vi "HFRR ADV v031 new software.vi"() -> ()   [LabVIEW 2025] (continued)
                    tunnel: w3949 -> [w3955 w3956 _ _ w3957 w3958 w3959 w3961 w3963 w3965 w3967 w3969 w3971 w3973 _]
                    tunnel: w3948 -> [_ _ _ _ _ _ _ _ _ _ _ _ _ _ _]
                    frame 0 {
                      "TITTLE" <- w3955
                    }
                    frame 1 {
                      "Sample ID" <- w3956
                    }
                    frame 2 {
                    }
                    frame 3 {
                    }
                    frame 4 {
                      "Test Date" <- w3957
                    }
                    frame 5 {
                      "Tested by" <- w3958
                    }
                    frame 6 {
                      n2895 = Fract/Exp String To Number(string=w3959) -> (number=→"Humidity before test 2":dbl)  [unwired: 3 in, 1 out]
                    }
                    frame 7 {
                      n2896 = Fract/Exp String To Number(string=w3961) -> (number=→"Temperature before test 2":dbl)  [unwired: 3 in, 1 out]
                    }
                    frame 8 {
                      n2897 = Fract/Exp String To Number(string=w3963) -> (number=→"Humidity after test 2":dbl)  [unwired: 3 in, 1 out]
                    }
                    frame 9 {
                      n2898 = Fract/Exp String To Number(string=w3965) -> (number=→"Temperature after test 2":dbl)  [unwired: 3 in, 1 out]
                    }
                    frame 10 {
                      n2899 = Fract/Exp String To Number(string=w3967) -> (number=→"MWSD 2":dbl)  [unwired: 3 in, 1 out]
                    }
                    frame 11 {
                      n2900 = Fract/Exp String To Number(string=w3969) -> (number=→"AVP 2":dbl)  [unwired: 3 in, 1 out]
                    }
                    frame 12 {
                      n2901 = Fract/Exp String To Number(string=w3971) -> (number=→"HCF 2":dbl)  [unwired: 3 in, 1 out]
                    }
                    frame 13 {
                      n2902 = Fract/Exp String To Number(string=w3973) -> (number=→"WS1.4 2":dbl)  [unwired: 3 in, 1 out]
                    }
                    frame 14, Default {
                    }
                  }
                }
              }
              frame #2 {
              }
            }
            n2903 = local write "OK Button 16"(FALSE ("OK Button 13")) -> ()
          }
        }
        n2904 = Index Array(array=w3618, index="Select Printer 3") -> (element=w3620:string)
        "Selected Printer" <- w3620
        n2905 = case shown="True" w3615 {
          frame False {
          }
          frame True {
            n2906 = flat-sequence {
              frame #0 {
              }
              frame #1 {
                n2907 = Wait (ms)(milliseconds to wait=u32 100) -> ()  [unwired: 1 out]
              }
              frame #2 {
                n2908 = local write "OK Button 16"(FALSE ("Print 3")) -> ()
              }
            }
          }
        }
        n2909 = case shown="True" "Print" {
          tunnel: w3620 -> [_ w3912]
          frame False {
          }
          frame True {
            (unwired) i16 6 ("width (-)")
            (unwired) "TESTED BY : "
            (unwired) "TESTED DATE :"
            (unwired) "SAMPLE ID : "
            (unwired) "SAMPLE DESIGN : "
            w3870 = "\r"
            w3887 = "\r"
            # "add image"
            n2910 = local read "Sample ID"() -> (w3860:string)
            n2911 = local read "Tested by"() -> (w3863:string)
            n2912 = local read "String 34"() -> (w3850:string)
            n2913 = local read "String 45"() -> (w3830:string)
            n2914 = local read "String 35"() -> (w3845:string)
            n2915 = local read "String 37"() -> (w3843:string)
            n2916 = local read "String 32"() -> (w3865:string)
            n2917 = local read "String 36"() -> (w3840:string)
            n2918 = local read "String 31"() -> (w3864:string)
            n2919 = local read "Test Date"() -> (w3861:string)
            n2920 = local read "String 33"() -> (w3866:string)
            n2921 = local read "String 38"() -> (w3836:string)
            n2922 = local read "String 39"() -> (w3833:string)
            n2923 = local write "Print"(FALSE ("Print FF")) -> ()
            n2924 = local read "S 39"() -> (w3848:string)
            n2925 = local read "S 38"() -> (w3855:string)
            n2926 = local read "Temperature before test 2"() -> (w3886:dbl)
            n2927 = local read "Temperature after test 2"() -> (w3876:dbl)
            n2928 = local read "Humidity before test 2"() -> (w3901:dbl)
            n2929 = local read "Humidity after test 2"() -> (w3885:dbl)
            n2930 = local read "MWSD 2"() -> (w3890:dbl)
            n2931 = local read "WS1.4 2"() -> (w3868:dbl)
            n2932 = Concatenate Strings("2)" ("string"), w3850) -> (w3851:string)
            n2933 = Concatenate Strings("3)" ("string"), w3848) -> (w3849:string)
            n2934 = Concatenate Strings("1)" ("string"), w3855) -> (w3854:string)
            n2935 = Concatenate Strings("4)" ("string"), w3845) -> (w3846:string)
            n2936 = Concatenate Strings("5)" ("string"), w3843) -> (w3842:string)
            n2937 = Concatenate Strings("6)" ("string"), w3840) -> (w3839:string)
            n2938 = Concatenate Strings("7)" ("string"), w3836) -> (w3837:string)
            n2939 = Concatenate Strings("8)" ("string"), w3833) -> (w3834:string)
            n2940 = local read "HCF 2"() -> (w3872:dbl)
            n2941 = local read "AVP 2"() -> (w3889:dbl)
            n2942 = local read "s.NO"() -> (w3831:string)
            n2943 = call <vilib>:"New Report.vi"("report type"=enum16{"Standard Report", "HTML"}."Standard Report") -> ("report out"=w3910:refnum<class "NI_report.lvclass">, "error out"=w3909:errorcluster)  [unwired: 13 in]
            n2944 = local read "TITTLE"() -> (w3862:string)
            n2945 = Concatenate Strings(w3887, w3830, w3831, w3887, w3865, w3860, w3887, w3864, w3861, w3887, w3866, w3863, w3887) -> (w3880:string)
            "test by" <- w3880
            n2946 = Number To Fractional String(number=w3886, width (-)=i16 6, precision (6)=i16 2) -> (F-format string=w3875:string)  [unwired: 1 in]
            n2947 = Number To Fractional String(number=w3885, width (-)=i16 6, precision (6)=i16 2) -> (F-format string=w3888:string)  [unwired: 1 in]
            n2948 = Number To Fractional String(number=w3901, width (-)=i16 6, precision (6)=i16 2) -> (F-format string=w3906:string)  [unwired: 1 in]
            n2949 = Number To Fractional String(number=w3890, width (-)=i16 6, precision (6)=i16 2) -> (F-format string=w3892:string)  [unwired: 1 in]
            n2950 = Number To Fractional String(number=w3876, width (-)=i16 6, precision (6)=i16 2) -> (F-format string=w3877:string)  [unwired: 1 in]
            n2951 = Number To Fractional String(number=w3889, width (-)=i16 6, precision (6)=i16 2) -> (F-format string=w3891:string)  [unwired: 1 in]
            n2952 = Number To Fractional String(number=w3872, width (-)=i16 6, precision (6)=i16 2) -> (F-format string=w3871:string)  [unwired: 1 in]
            n2953 = Number To Fractional String(number=w3868, precision (6)=i16 2) -> (F-format string=w3867:string)  [unwired: 2 in]
            n2954 = call-dynamic "Set Report Header Text.vi"("report in"=w3910, "center header text"=w3862, "error in (no error)"=w3909) -> ("report out"=w3881:refnum<class "NI_report.lvclass">, "error out"=w3882:errorcluster)  [unwired: 11 in]
            n2955 = Concatenate Strings(w3870, w3854, w3906, w3870, w3851, w3875, w3870, w3849, w3888, w3870, w3846, w3877, w3870, w3842, w3892, w3870, w3839, w3891, w3870, w3837, w3871, w3870, w3834, w3867) -> (w3858:string)
            "export 2" <- w3858
            n2956 = call-poly <vilib>:"Append Report Text.vi"("report in"=w3881, "text"=w3880, "error in (no error)"=w3882) -> ("report out"=w3884:refnum<class "NI_report.lvclass">, "error out"=w3883:errorcluster)  [unwired: 9 in, 2 out]
            n2957 = local read "test by"() -> (w3857:string)
            n2958 = local read "TITTLE"() -> (w3859:string)
            n2959 = call-poly <vilib>:"Append Report Text.vi"("report in"=w3884, "error in (no error)"=w3883) -> ("report out"=w3905:refnum<class "NI_report.lvclass">, "error out"=w3903:errorcluster)  [unwired: 10 in, 2 out]
            n2960 = Concatenate Strings(w3859, w3858, w3857) -> (→"output":string)
            n2961 = call-poly <vilib>:"Append Report Text.vi"("report in"=w3905, "text"=w3858, "error in (no error)"=w3903) -> ("report out"=w3904:refnum<class "NI_report.lvclass">, "error out"=w3902:errorcluster)  [unwired: 9 in, 2 out]
            n2962 = call-dynamic "Print Report.vi"("report in"=w3904, "printer name (default)"=w3912, "error in (no error)"=w3902) -> ("report out"=w3914:refnum<class "NI_report.lvclass">, "error out"=w3915:errorcluster)  [unwired: 11 in]
            n2963 = call-dynamic "Dispose Report.vi"("report in"=w3914, "error in (no error)"=w3915) -> ()  [unwired: 13 in, 1 out]
          }
        }
        n2964 = case shown="True" "Print 2" {
          frame False {
          }
          frame True {
            n2965 = flat-sequence {
              frame #0 {
                n2966 = local read "s.NO"() -> (→"s.NO 2":string)
                n2967 = Wait (ms)(milliseconds to wait=u32 20) -> ()  [unwired: 1 out]
                n2968 = local read "Sample ID  3"() -> (→"Sample ID  6":string)
                n2969 = local read "Sample ID  4"() -> (→"Sample ID  7":string)
                n2970 = local read "Sample ID"() -> (→"Sample ID  2":string)
                n2971 = local read "Tested by"() -> (→"Tested by 2":string)
                n2972 = local read "Test Date"() -> (→"Test Date 2":string)
                n2973 = local read "Humidity after test 3"() -> (→"Humidity after test 4":dbl)
                n2974 = local read "Ref A Test Date :"() -> (→"TITTLE 4":string)
                n2975 = local read "Temperature before test 3"() -> (w3737:dbl)
                n2976 = local read "Temperature before test 3"() -> (→"Temperature after test 5":dbl)
                n2977 = local read "Temperature after test 3"() -> (→"Temperature after test 4":dbl)
                n2978 = local read "Humidity before test 3"() -> (→"Humidity before test 4":dbl)
                n2979 = local write "Temperature before test 3"(w3737) -> ()
                n2980 = local read "image data"() -> (w3728:T16)
                n2981 = String To Path(string="C:\\LAB-IQ\\im\\Temp_resized.jpg") -> (path=w3729:path)
                "path 2" <- w3729
                n2982 = call <vilib>:"Write JPEG File.vi"("image data"=w3728, "path to JPEG file"=w3729) -> ()  [unwired: 8 in, 2 out]
                "Ref A Test Date :" <- "Ref A Test Date :"
                "Ref B Test Date :" <- "Ref B Test Date :"
                "Ref B Scar Value :" <- "Ref B Scar Value :"
                "Ref A Scar Value :" <- "Ref A Scar Value :"
              }
              frame #1 {
                (unwired) HTML_Report_Image_Alignment."MIDDLE" ("alignment (default)")
                w3765 = u16 0 items=["portrait", "landscape"] ("orientation (portrait)")
                (unwired) HTML_Report_Image_Alignment."ABSMIDDLE" ("alignment (default)")
                (unwired) "TESTED BY : "
                (unwired) "TESTED DATE :"
                (unwired) "SAMPLE ID : "
                (unwired) "SAMPLE DESIGN : "
                w3798 = "\r"
                # "add image"
                n2983 = Wait (ms)(milliseconds to wait=u32 20) -> ()  [unwired: 1 out]
                n2984 = local read "Sample ID  2"() -> (w3791:string)
                n2985 = local read "Wear Scar X"() -> (w3763:dbl)
                "Length ( microns ) 2" <- w3763
                n2986 = local read "Wear Scar Y"() -> (w3762:dbl)
                "Wear Scar Y ( microns ) :" <- w3762
                n2987 = local read "Test Date 2"() -> (w3792:string)
                n2988 = local read "Tested by 2"() -> (w3793:string)
                n2989 = local read "String 46"() -> (w3789:string)
                n2990 = local read "String 48"() -> (w3795:string)
                n2991 = local read "String 47"() -> (w3794:string)
                n2992 = local read "String 49"() -> (w3796:string)
                n2993 = local read "String 10"() -> (w3749:string)
                n2994 = local read "s.NO 2"() -> (w3790:string)
                n2995 = Add(x=w3763, y=w3762) -> (x+y=w3761:dbl)
                n2996 = call <vilib>:"New Report.vi"("report type"=enum16{"Standard Report", "HTML"}."HTML") -> ("report out"=w3769:refnum<class "NI_report.lvclass">, "error out"=w3767:errorcluster)  [unwired: 13 in]
                n2997 = Concatenate Strings(w3798, w3789, w3790, w3798, w3795, w3791, w3798, w3794, w3792, w3798, w3796, w3793, w3798) -> (→"test by 2":string)
                n2998 = Concatenate Strings("C:\\LAB-IQ\\Data\\" ("string"), w3749, ".jpg" ("string")) -> ()  [unwired: 1 out]
                n2999 = Divide(x=w3761, y=2.0) -> (x/y=→"Mean Wear ( microns) :":dbl)
                n3000 = call-dynamic "Set Report Orientation.vi"("report in"=w3769, "orientation (portrait)"=w3765, "error in (no error)"=w3767) -> ("report out"=w3768:refnum<class "NI_report.lvclass">, "error out"=w3766:errorcluster)  [unwired: 11 in]
                n3001 = for {
                  N: 5 -> [_]
                  tunnel: w3768 -> [w3819]
                  tunnel: [w3818] -> w3747
                  tunnel: w3766 -> [w3817]
                  tunnel: [w3816] -> w3746
                  n3002 = call-dynamic "Set Report Tab Width.vi"("report in"=w3819, "error in (no error)"=w3817) -> ("report out"=w3818:refnum<class "NI_report.lvclass">, "error out"=w3816:errorcluster)  [unwired: 12 in]
                }
                n3003 = local read "TITTLE"() -> (w3764:string)
                n3004 = call-dynamic "Set Report Header Text.vi"("report in"=w3747, "center header text"=w3764, "error in (no error)"=w3746) -> ("report out"=w3785:refnum<class "NI_report.lvclass">, "error out"=w3784:errorcluster)  [unwired: 11 in]
                n3005 = for {
                  N: 1 -> [_]
                  tunnel: [w3823] -> w3771
                  tunnel: [w3822] -> w3770
                  tunnel: w3785 -> [w3821]
                  tunnel: w3784 -> [w3820]
                  n3006 = call-dynamic "New Report Line.vi"("report in"=w3821, "error in (no error)"=w3820) -> ("report out"=w3823:refnum<class "NI_report.lvclass">, "error out"=w3822:errorcluster)  [unwired: 12 in]
                }
                n3007 = for {
                  N: 2 -> [_]
                  tunnel: [w3815] -> w3777
                  tunnel: [w3814] -> w3776
                  tunnel: w3771 -> [w3813]
                  tunnel: w3770 -> [w3812]
                  n3008 = call-dynamic "New Report Line.vi"("report in"=w3813, "error in (no error)"=w3812) -> ("report out"=w3815:refnum<class "NI_report.lvclass">, "error out"=w3814:errorcluster)  [unwired: 12 in]
                }
                n3009 = for {
                  N: 25 -> [_]
                  tunnel: w3777 -> [w3811]
                  tunnel: w3776 -> [w3809]
                  tunnel: [w3810] -> w3780
                  tunnel: [w3808] -> w3779
                  n3010 = call-dynamic "Set Report Tab Width.vi"("report in"=w3811, "error in (no error)"=w3809) -> ("report out"=w3810:refnum<class "NI_report.lvclass">, "error out"=w3808:errorcluster)  [unwired: 12 in]
                }
                n3011 = control-ref of="Tab Control 9"() -> (w3775:refnum<vi>)
                n3012 = call-dynamic "Append Control Image to Report.vi"("report in"=w3780, "alignment (default)"=HTML_Report_Image_Alignment."ABSMIDDLE", "ctrl reference"=w3775, "error in (no error)"=w3779) -> ("report out"=w3774:refnum<class "NI_report.lvclass">, "error out"=w3773:errorcluster)  [unwired: 8 in, 2 out]
                n3013 = for {
                  N: 3 -> [_]
                  tunnel: [w3807] -> w3758
                  tunnel: [w3806] -> w3757
                  tunnel: w3774 -> [w3805]
                  tunnel: w3773 -> [w3804]
                  n3014 = call-dynamic "New Report Line.vi"("report in"=w3805, "error in (no error)"=w3804) -> ("report out"=w3807:refnum<class "NI_report.lvclass">, "error out"=w3806:errorcluster)  [unwired: 12 in]
                }
                n3015 = for {
                  N: 100 -> [_]
                  tunnel: w3758 -> [w3803]
                  tunnel: w3757 -> [w3801]
                  tunnel: [w3802] -> w3754
                  tunnel: [w3800] -> w3752
                  n3016 = call-dynamic "Set Report Tab Width.vi"("report in"=w3803, "error in (no error)"=w3801) -> ("report out"=w3802:refnum<class "NI_report.lvclass">, "error out"=w3800:errorcluster)  [unwired: 12 in]
                }
                n3017 = String To Path(string="C:\\LAB-IQ\\im\\Temp_resized.jpg") -> (path=w3744:path)
                n3018 = call-poly <vilib>:"Append Image to Report.vi"("report in"=w3754, "path or URL of image"=w3744, "error in (no error)"=w3752) -> ("report out"=w3753:refnum<class "NI_report.lvclass">, "error out"=w3751:errorcluster)  [unwired: 9 in, 2 out]
                n3019 = call-poly <vilib>:"Open HTML Report in Browser.vi"("report in"=w3753, "error in (no error)"=w3751) -> ("report out"=w3788:refnum<class "NI_report.lvclass">, "error out"=w3787:errorcluster)  [unwired: 11 in, 1 out]
                n3020 = call-dynamic "Dispose Report.vi"("report in"=w3788, "error in (no error)"=w3787) -> ()  [unwired: 13 in, 1 out]
              }
              frame #2 {
              }
              frame #3 {
                n3021 = disable-structure shown="Disabled" {
                  frame Disabled {
                    n3022 = local read "String 10"() -> (w3828:string)
                    n3023 = Concatenate Strings("C:\\LAB-IQ-NXT\\Data\\" ("string"), w3828, ".jpg" ("string")) -> (w3826:string)
                    n3024 = String To Path(string=w3826) -> (path=w3825:path)
                    n3025 = Delete(path (use dialog)=w3825) -> ()  [unwired: 4 in, 3 out]
                  }
                  frame Enabled {
                  }
                }
                n3026 = local write "Print 2"(FALSE ("Print")) -> ()
              }
            }
          }
        }
      }
    }
    n3027 = Wait (ms)(milliseconds to wait=u32 50) -> ()  [unwired: 1 out]
    n3028 = Wait (ms)(milliseconds to wait=u32 50) -> ()  [unwired: 1 out]
    n3029 = local read "Quit"() -> (w2172:bool)
  }
  n3030 = VISA Close(VISA resource name=w41, error in (no error)=w40) -> ()  [unwired: 1 out]
  n3031 = while {
    stop <- w3979 stop-if-true
    n3032 = local read "Auto Start Test"() -> (w3977:bool)
    n3033 = local read "RUN"() -> (w3976:bool)
    n3034 = Wait (ms)(milliseconds to wait=u32 1000) -> ()  [unwired: 1 out]
    n3035 = Or(x=w3976, y=w3977) -> (x .or. y?=w3975:bool)
    n3036 = case shown="True" w3975 {
      frame False {
      }
      frame True {
        n3037 = local read "LVDT STROKE Actual"() -> (w3980:dbl)
        n3038 = In Range and Coerce(upper limit=1.2, x=w3980, lower limit=0.6) -> (In Range?=w3983:bool)  [unwired: 1 out]
        n3039 = call-poly <vilib>:"Random Number (Range).vi"("lower bound (0)"=0.998 ("upper bound (100)"), "upper bound (100)"=1.003) -> ("number"=w3981:dbl)  [unwired: 9 in]
        n3040 = case shown="True" w3983 {
          tunnel: [w3988 w3989] -> w3982
          tunnel: w3981 -> [_ w3989]
          tunnel: w3980 -> [w3988 _]
          frame False {
          }
          frame True {
          }
        }
        "LVDT STROKE DISPLAY" <- w3982
      }
    }
    n3041 = local read "Quit"() -> (w3979:bool)
  }
  n3042 = while {
    tunnel: [w4006] -> w49
    shift-right: [w3999] -> _
    shift-left: 0.0 -> [w4002]
    shift-right: [w3998] -> _
    shift-left: 0.0 -> [w4001]
    shift-right: [w3997] -> _
    shift-left: 100.0 ("vc_cmd") -> [w4000]
    stop <- w4006 stop-if-true
    # "PID LOGIC"
    n3043 = local read "run test Calibration"() -> (w3994:bool)
    n3044 = local read "RUN"() -> (w4004:bool)
    n3045 = local read "Auto Start Temp"() -> (w3995:bool)
    n3046 = local read "Auto Start Test"() -> (w4003:bool)
    n3047 = local read "START TEMP"() -> (w3993:bool)
    n3048 = And(x=w3995, y=w4003) -> (x .and. y?=w3996:bool)
    n3049 = Or(x=w4004, y=w3996) -> (x .or. y?=w4005:bool)
    n3050 = And(x=w4005, y=w3993) -> (x .and. y?=w3992:bool)
    n3051 = And(x=w3994, y=w3993) -> (x .and. y?=w3991:bool)
    n3052 = Or(x=w3991, y=w3992) -> (x .or. y?=w3990:bool)
    n3053 = Wait (ms)(milliseconds to wait="milliseconds to wait") -> ()  [unwired: 1 out]
    n3054 = case shown="True" w3990 {
      tunnel: [400.0 ("out_vc_cmd") w4025] -> w3997
      tunnel: [w4009 w4027] -> w3998
      tunnel: [w4009 w4026] -> w3999
      tunnel: w4002 -> [_ w4016]
      tunnel: w4001 -> [_ w4015]
      tunnel: w4000 -> [_ w4014]
      tunnel: w3994 -> [_ w4010]
      frame False {
        w4009 = 0.0 ("error_out")
      }
      frame True {
        n3055 = case shown="True" w4010 {
          tunnel: [w4034 1.0] -> w4012
          frame False {
            n3056 = local read "Set Strk"() -> (w4033:dbl)
            n3057 = Add(x=w4033, y="Add up Stroke") -> (x+y=w4034:dbl)
          }
          frame True {
          }
        }
        n3058 = local read "LVDT STROKE"() -> (w4011:dbl)
        n3059 = formula code="// Zero-Hardcode Explicit Positional-Form PID Engine\n// Inputs: target_stroke, measured_stroke, dt, prev_error, integral_accumulator_in, prev_vc_cmd\n//         kp, ki, kd, max_step_change, max_amplitude, min_amplitude, startup_cmd\n// Outputs: vc_cmd, error_out, out_error, integral_accumulator_out, out_vc_cmd\n\n// 1. Calculate Tracking Error\nfloat current_error = target_stroke - measured_stroke;\nerror_out = current_error;\n\n// 2. Compute Proportional Term\nfloat p_term = kp * current_error;\n\n// 3. Compute Derivative Term\nfloat d_term = 0.0;\nif (dt > 0.0) {\n    d_term = kd * ((current_error - prev_error) / dt);\n}\n\n// 4. Update and Accumulate Integral Term\nfloat current_integral = integral_accumulator_in + (current_error * dt);\nfloat i_term = ki * current_integral;\n\n// 5. Calculate Ideal Target Command (Anchored by startup baseline)\nfloat ideal_command = startup_cmd + p_term + i_term + d_term;\n\n// 6. Apply Loop Rate Limiting FIRST \n// (Forces the command to climb gradually from prev_vc_cmd instead of jumping straight to max)\nfloat raw_adjustment = ideal_command - prev_vc_cmd;\n\nif (raw_adjustment > max_step_change) {\n    raw_adjustment = max_step_change;\n} else if (raw_adjustment < -max_step_change) {\n    raw_adjustment = -max_step_change;\n}\n\nfloat next_vc_cmd = prev_vc_cmd + raw_adjustment;\n\n// 7. Anti-Windup Protection & Final Output Safety Safeguard Clamping\n// (Back-calculating based on what we are ACTUALLY outputting)\nif (next_vc_cmd > max_amplitude) {\n    float excess = next_vc_cmd - max_amplitude;\n    if (ki > 0.0) {\n        current_integral -= excess / ki;\n    }\n    next_vc_cmd = max_amplitude;\n} else if (next_vc_cmd < min_amplitude) {\n    float excess = next_vc_cmd - min_amplitude;\n    if (ki > 0.0) {\n        current_integral -= excess / ki;\n    }\n    next_vc_cmd = min_amplitude;\n}\n\n// 8. Map to Shift Registers for memory persistence\nvc_cmd = next_vc_cmd;\nout_error = current_error;                   \nintegral_accumulator_out = current_integral;  \nout_vc_cmd = next_vc_cmd;"("target_stroke"=w4012, "measured_stroke"=w4011, "dt"="dt", "integral_accumulator_in"=w4015, "prev_error"=w4016, "prev_vc_cmd"=w4014, "kp"="kp", "ki"="ki", "kd"="kd", "max_step_change"="max_step_change", "max_amplitude"="max_amplitude", "min_amplitude"="min_amplitude", "startup_cmd"="startup_cmd") -> ("vc_cmd"=w4031:dbl, "out_error"=w4026:dbl, "integral_accumulator_out"=w4027:dbl, "out_vc_cmd"=w4025:dbl)  [unwired: 1 out]
        "output Vpp" <- w4031
        n3060 = Number To Fractional String(number=w4031, precision (6)=i16 1) -> (F-format string=w4029:string)  [unwired: 2 in]
        n3061 = Concatenate Strings("DAC;" ("string"), w4029) -> (w4013:string)
        n3062 = local write "Due Write"(w4013) -> ()
        "prev_error" <- w4016
        "integral_accumulator_in" <- w4015
        "prev_vc_cmd" <- w4014
      }
    }
    n3063 = local read "Quit"() -> (w4006:bool)
  }
  n3064 = Or(x=w45, y=w44) -> (x .or. y?=w46:bool)
  n3065 = Or(x=w42, y=w46) -> (x .or. y?=w51:bool)
  n3066 = control-ref of="new picture"() -> ()  [unwired: 1 out]
  n3067 = Or(x=w54, y=w51) -> (x .or. y?=w48:bool)
  n3068 = Or(x=w48, y=w49) -> (x .or. y?=w43:bool)
  n3069 = while {
    tunnel: [w4036] -> w53
    i -> [w4043]
    stop <- w4036 stop-if-true
    n3070 = local read "Quit"() -> (w4036:bool)
    n3071 = Equal To 0?(x=w4043) -> (x = 0?=w4041:bool)
    n3072 = call "Elapsed Time3"("Time Target (s)"=45.0, "Auto Reset"=TRUE) -> ("Time has Elapsed"=w4040:bool)  [unwired: 10 in, 7 out]
    n3073 = Wait (ms)(milliseconds to wait=u32 50) -> ()  [unwired: 1 out]
    n3074 = Or(x=w4040, y=w4041) -> (x .or. y?=w4042:bool)
    n3075 = case shown="True" w4042 {
      frame False {
      }
      frame True {
        n3076 = call <vilib>:"System Exec.vi"("run minimized? (F)"=TRUE, "error in (no error)"="error in (no error)", "command line"="powercfg.exe -change -monitor-timeout-ac 0") -> ("error out"=w4054:errorcluster)  [unwired: 5 in, 3 out]
        n3077 = call <vilib>:"System Exec.vi"("run minimized? (F)"=TRUE, "error in (no error)"=w4054, "command line"="powercfg.exe -change -disk-timeout-ac 0") -> ("error out"=w4053:errorcluster)  [unwired: 5 in, 3 out]
        n3078 = call <vilib>:"System Exec.vi"("run minimized? (F)"=TRUE, "error in (no error)"=w4053, "command line"="powercfg.exe -change -standby-timeout-ac 0") -> ("error out"=w4052:errorcluster)  [unwired: 5 in, 3 out]
        n3079 = call <vilib>:"System Exec.vi"("run minimized? (F)"=TRUE, "error in (no error)"=w4052, "command line"="powercfg.exe -change -hibernate-timeout-ac 0") -> ("error out"=w4051:errorcluster)  [unwired: 5 in, 3 out]
        n3080 = call <vilib>:"Simple Error Handler.vi"("error in (no error)"=w4051) -> ("error out"=w4057:errorcluster)  [unwired: 4 in, 4 out]
        n3081 = call <vilib>:"Clear Errors.vi"("error in (no error)"=w4057) -> ("error out"=→"error out":errorcluster)  [unwired: 5 in, 1 out]
      }
    }
  }
  n3082 = Compound Arithmetic op=OR(w56, w43, w53) -> (w55:bool)
  n3083 = flat-sequence {
    tunnel: w55 -> [_]
    tunnel: [w4059] -> w25
    tunnel: w25 -> [_]
    frame #0 {
      n3084 = call "CLOSE CONNECTION.vi"() -> ("error out"=w4059:errorcluster)  [unwired: 11 in]
    }
    frame #1 {
      n3085 = Quit LabVIEW(quit? (T)=TRUE) -> ()
      n3086 = local write "Quit"(FALSE ("EXIT")) -> ()
    }
  }
  n3087 = property on="Heater Button" class="Bool (strict)"("Visible"=TRUE) -> ()  [unwired: 2 in, 2 out]
  n3088 = while {
    tunnel: [w4066] -> _
    i -> [w4066]
    stop <- w4062 stop-if-true
    # "Langauage selection"
    n3089 = Equal?(x="Lan flag", y=22.0) -> ()  [unwired: 1 out]
    n3090 = disable-structure shown="Disabled" {
      frame Disabled {
        n3091 = stacked-sequence {
          frame #0 {
            n3092 = case shown="\"Russian\"" "Language Selection" {
              tunnel: [0 1] -> w4068
              frame "English", Default {
              }
              frame "Russian" {
              }
            }
            n3093 = for {
              N: 130 -> [_]
              tunnel: "Table" -> [w4077]
              tunnel: w4068 -> [w4076]
              i -> [w4075]
              n3094 = Index Array(array=w4077, index (row)=w4075, index (col)=w4076) -> (element=w4074:string)
              n3095 = case shown="1" w4075 {
                tunnel: w4074 -> [w4078 w4079 _ w4080 w4081 w4082 w4083 w4084 w4085 w4086 w4087 w4088 w4089 w4090 w4091 w4092 w4093 w4094 w4095 w4096 w4097 w4098 w4099 w4100 w4101 w4102 w4103 w4104 w4105 _ _ w4106 w4107 w4108 w4109 w4110 w4111 w4120 w4127 w4134 w4141 w4145 w4148 w4151 w4153 w4155 w4156 w4157 w4158 w4159 w4160 w4161 w4162 w4163 w4164 w4165 w4166 w4167 w4168 w4169 w4170 w4171 w4172 w4173 w4174 w4175 w4176 w4177 w4178 w4179 w4180 w4181 w4182 w4183 w4184 w4185 w4186 w4187 w4188 w4189 w4190 w4191 w4192 w4193 w4194 w4195 w4196 w4197 w4198 w4199 w4200 w4201 w4202 w4203 w4204 w4205 w4206 w4207 w4208 w4209 w4210 w4211 w4212 w4213 w4214 _ w4215 w4216 w4217 w4218 w4219 w4220 w4221 w4222 w4223 w4224 w4225 w4226 w4227 _ w4228 w4229 w4230 w4231 w4232 w4233 _]
                frame 0 {
                  n3096 = local write "S"(w4078) -> ()
                }
                frame 1 {
                  n3097 = local write "S 2"(w4079) -> ()
                }
                frame 2 {
                }
                frame 3 {
                  n3098 = local write "S 4"(w4080) -> ()
                }
                frame 4 {
                  n3099 = property on="FILE" class="Str"("Caption.Text"=w4081) -> ()  [unwired: 2 in, 2 out]
                }
                frame 5 {
                  n3100 = property on="Fuel Discription :" class="Str"("Caption.Text"=w4082) -> ()  [unwired: 2 in, 2 out]
                }
                frame 6 {
                  n3101 = property on="Remarks :" class="Str"("Caption.Text"=w4083) -> ()  [unwired: 2 in, 2 out]
                }
                frame 7 {
                  n3102 = property on="Save & Continue" class="Bool (strict)"("Boolean Text.Text"=w4084) -> ()  [unwired: 2 in, 2 out]
                }
                frame 8 {
                }
                frame 9 {
                  n3103 = property on="Set Hz" class="DigNum (strict)"("Caption.Text"=w4086) -> ()  [unwired: 2 in, 2 out]
                }
                frame 10 {
                }
                frame 11 {
                  n3104 = property on="NORMAL LOAD" class="DigNum (strict)"("Caption.Text"=w4088) -> ()  [unwired: 2 in, 2 out]
                }
                frame 12 {
                }
                frame 13 {
                  n3105 = property on="Set Temp" class="DigNum (strict)"("Caption.Text"=w4090) -> ()  [unwired: 2 in, 2 out]
                }
                frame 14 {
                  n3106 = local write "S 15"(w4091) -> ()
                }
                frame 15 {
                  n3107 = property on="Set Rh" class="DigNum (strict)"("Caption.Text"=w4092) -> ()  [unwired: 2 in, 2 out]
                }
                frame 16 {
                }
                frame 17 {
                  n3108 = local write "S 18"(w4094) -> ()
                }
                frame 18 {
                  "String 17" <- w4095
                }
                frame 19 {
                  n3109 = property on="test time" class="DigNum (strict)"("Caption.Text"=w4096) -> ()  [unwired: 2 in, 2 out]
                }
                frame 20 {
                  "String 18" <- w4097
                  "String 22" <- w4097
                }
                frame 21 {
                  n3110 = property on="Elapsed time" class="DigNum (strict)"("Caption.Text"=w4098) -> ()  [unwired: 2 in, 2 out]
                }
                frame 22 {
                  n3111 = property on="Samplingtime 2" class="DigNum (strict)"("Caption.Text"=w4099) -> ()  [unwired: 2 in, 2 out]
                }
                frame 23 {
                  "String 21" <- w4100
                }
                frame 24 {
                  n3112 = property on="Countdown" class="DigNum (strict)"("Caption.Text"=w4101) -> ()  [unwired: 2 in, 2 out]
                }
                frame 25 {
                  n3113 = property on="Countdown 2" class="DigNum (strict)"("Caption.Text"=w4102) -> ()  [unwired: 2 in, 2 out]
                }
                frame 26 {
                  n3114 = property on="Engage" class="Bool (strict)"("Boolean Text.Text"=w4103) -> ()  [unwired: 2 in, 2 out]
                }
                frame 27 {
                  n3115 = property on="Boolean  4" class="Bool (strict)"("Boolean Text.Text"=w4104) -> ()  [unwired: 2 in, 2 out]
                }
                frame 28 {
                  n3116 = property on="Test \nStatus" class="Bool (strict)"("Boolean Text.Text"=w4105) -> ()  [unwired: 2 in, 2 out]
                }
                frame 29 {
                }
                frame 30 {
                }
                frame 31 {
                }
                frame 32 {
                  n3117 = property on="RSTCOF" class="Bool"("Boolean Text.Text"=w4107) -> ()  [unwired: 2 in, 2 out]
                  n3118 = property on="RST FF" class="Bool"("Boolean Text.Text"=w4107) -> ()  [unwired: 2 in, 2 out]
                  n3119 = property on="RST TEMP" class="Bool"("Boolean Text.Text"=w4107) -> ()  [unwired: 2 in, 2 out]
                  n3120 = property on="RSTV1 3" class="Bool"("Boolean Text.Text"=w4107) -> ()  [unwired: 2 in, 2 out]
                  n3121 = property on="rstv2" class="Bool"("Boolean Text.Text"=w4107) -> ()  [unwired: 2 in, 2 out]
                  n3122 = property on="RSTV1 2" class="Bool"("Boolean Text.Text"=w4107) -> ()  [unwired: 2 in, 2 out]
                  n3123 = property on="RST CP" class="Bool"("Boolean Text.Text"=w4107) -> ()  [unwired: 2 in, 2 out]
                }
                frame 33 {
                  "S 61" <- w4108
                }
                frame 34 {
                  "String 23" <- w4109
                }
                frame 35 {
                  n3124 = property on="Rh Before" class="DigNum (strict)"("Caption.Text"=w4110) -> ()  [unwired: 2 in, 2 out]
                }
                frame 36 {
                  n3125 = Match Pattern(string=w4111, regular expression=",") -> (before substring=→"bs":string, after substring=→"as":string)  [unwired: 1 in, 2 out]
                  n3126 = property on="Rh After" class="DigNum (strict)"("Caption.Text"=w4111) -> ()  [unwired: 2 in, 2 out]
                }
                frame 37 {
                  n3127 = Match Pattern(string=w4120, regular expression=",") -> (before substring=w4119:string, after substring=w4118:string)  [unwired: 1 in, 2 out]
                  "bs" <- w4119
                  "as" <- w4118
                  n3128 = Concatenate Strings(w4119, w4118) -> (w4115:string)
                  n3129 = property on="Humidity before test 2" class="DigNum (strict)"("Caption.Text"=w4115) -> ()  [unwired: 2 in, 2 out]
                  n3130 = Concatenate Strings(w4115, "=" ("string")) -> (w4116:string)
                  n3131 = local write "S 38"(w4116) -> ()
                }
                frame 38 {
                  n3132 = Match Pattern(string=w4127, regular expression=",") -> (before substring=w4126:string, after substring=w4125:string)  [unwired: 1 in, 2 out]
                  "bs" <- w4126
                  "as" <- w4125
                  n3133 = Concatenate Strings(w4126, w4125) -> (w4122:string)
                  n3134 = property on="Humidity after test 2" class="DigNum (strict)"("Caption.Text"=w4122) -> ()  [unwired: 2 in, 2 out]
                  n3135 = Concatenate Strings(w4122, "=" ("string")) -> (w4124:string)
                  n3136 = local write "S 39"(w4124) -> ()
                }
                frame 39 {
                  n3137 = Match Pattern(string=w4134, regular expression=",") -> (before substring=w4133:string, after substring=w4132:string)  [unwired: 1 in, 2 out]
                  "bs" <- w4133
                  "as" <- w4132
                  n3138 = Concatenate Strings(w4133, w4132) -> (w4129:string)
                  n3139 = property on="Temperature before test 2" class="DigNum (strict)"("Caption.Text"=w4129) -> ()  [unwired: 2 in, 2 out]
                  n3140 = Concatenate Strings(w4129, "=" ("string")) -> (→"String 34":string)
                }
                frame 40 {
                  n3141 = Match Pattern(string=w4141, regular expression=",") -> (before substring=w4140:string, after substring=w4139:string)  [unwired: 1 in, 2 out]
                  "bs" <- w4140
                  "as" <- w4139
                  n3142 = Concatenate Strings(w4140, w4139) -> (w4136:string)
                  n3143 = property on="Temperature after test 2" class="DigNum (strict)"("Caption.Text"=w4136) -> ()  [unwired: 2 in, 2 out]
                  n3144 = Concatenate Strings(w4136, "=" ("string")) -> (→"String 35":string)
                  n3145 = property on="Temperature after test" class="DigNum (strict)"("Caption.Text"=w4136) -> ()  [unwired: 2 in, 2 out]
                }
                frame 41 {
                  n3146 = property on="AVP 2" class="DigNum (strict)"("Caption.Text"=w4145) -> ()  [unwired: 2 in, 2 out]
                  n3147 = Concatenate Strings(w4145, "=" ("string")) -> (→"String 36":string)
                }
                frame 42 {
                  n3148 = property on="MWSD 2" class="DigNum (strict)"("Caption.Text"=w4148) -> ()  [unwired: 2 in, 2 out]
                  n3149 = Concatenate Strings(w4148, "=" ("string")) -> (→"String 37":string)
                }
                frame 43 {
                  n3150 = property on="HCF 2" class="DigNum (strict)"("Caption.Text"=w4151) -> ()  [unwired: 2 in, 2 out]
                  n3151 = Concatenate Strings(w4151, "=" ("string")) -> (→"String 38":string)
                }
                frame 44 {
                  n3152 = Concatenate Strings(w4153, "=" ("string")) -> (→"String 39":string)
                  n3153 = property on="WS1.4 2" class="DigNum (strict)"("Caption.Text"=w4153) -> ()  [unwired: 2 in, 2 out]
                }
                frame 45 {
                }
                frame 46 {
                  n3154 = local write "S 47"(w4156) -> ()
                }
                frame 47 {
                  n3155 = local write "S 48"(w4157) -> ()
                }
                frame 48 {
                  n3156 = local write "S 49"(w4158) -> ()
                }
                frame 49 {
                  n3157 = local write "S 50"(w4159) -> ()
                }
                frame 50 {
                  n3158 = local write "S 51"(w4160) -> ()
                }
                frame 51 {
                  n3159 = local write "S 52"(w4161) -> ()
                }
                frame 52 {
                  n3160 = local write "S 53"(w4162) -> ()
                }
                frame 53 {
                  n3161 = local write "S 54"(w4163) -> ()
                }
                frame 54 {
                  n3162 = local write "S 55"(w4164) -> ()
                }
                frame 55 {
                  n3163 = local write "S 56"(w4165) -> ()
                }
                frame 56 {
                  n3164 = local write "S 57"(w4166) -> ()
                }
                frame 57 {
                  n3165 = local write "S 58"(w4167) -> ()
                }
                frame 58 {
                  n3166 = local write "S 59"(w4168) -> ()
                }
                frame 59 {
                  n3167 = local write "S 60"(w4169) -> ()
                }
                frame 60 {
                  n3168 = local write "S 62"(w4170) -> ()
                }
                frame 61 {
                  n3169 = local write "S 63"(w4171) -> ()
                }
                frame 62 {
                  n3170 = local write "S 64"(w4172) -> ()
                }
                frame 63 {
                  n3171 = local write "S 65"(w4173) -> ()
                }
                frame 64 {
                  n3172 = local write "S 66"(w4174) -> ()
                }
                frame 65 {
                  n3173 = local write "S 67"(w4175) -> ()
                }
                frame 66 {
                  n3174 = local write "S 68"(w4176) -> ()
                }
                frame 67 {
                  n3175 = local write "S 69"(w4177) -> ()
                }
                frame 68 {
                  n3176 = local write "S 70"(w4178) -> ()
                }
                frame 69 {
                  n3177 = local write "S 71"(w4179) -> ()
                }
                frame 70 {
                  n3178 = local write "S 72"(w4180) -> ()
                }
                frame 71 {
                  n3179 = local write "S 73"(w4181) -> ()
                }
                frame 72 {
                  n3180 = local write "S 74"(w4182) -> ()
                }
                frame 73 {
                  n3181 = local write "S 75"(w4183) -> ()
                }
                frame 74 {
                  n3182 = local write "S 76"(w4184) -> ()
                }
                frame 75 {
                  n3183 = local write "S 77"(w4185) -> ()
                }
                frame 76 {
                  n3184 = local write "S 78"(w4186) -> ()
                }
                frame 77 {
                  n3185 = local write "S 79"(w4187) -> ()
                }
                frame 79 {
                  n3186 = property on="Sample Temperature ( °C )" class="XYGraph (strict)"("Y Scale.Name Label.Text"=w4188) -> ()  [unwired: 2 in, 2 out]
                }
                frame 80 {
                  n3187 = local write "S 81"(w4189) -> ()
                  n3188 = property on="Humidity ( %RH )" class="XYGraph (strict)"("Y Scale.Name Label.Text"=w4189) -> ()  [unwired: 2 in, 2 out]
                }
                frame 78 {
                  n3189 = property on="Air Temperature  ( °C )" class="XYGraph (strict)"("X Scale.Name Label.Text"=w4190) -> ()  [unwired: 2 in, 2 out]
                  n3190 = property on="Humidity ( %RH )" class="XYGraph (strict)"("X Scale.Name Label.Text"=w4190) -> ()  [unwired: 2 in, 2 out]
                  n3191 = property on="Sample Temperature ( °C )" class="XYGraph (strict)"("X Scale.Name Label.Text"=w4190) -> ()  [unwired: 2 in, 2 out]
                  n3192 = property on="Coefficient Of Friction" class="XYGraph (strict)"("X Scale.Name Label.Text"=w4190) -> ()  [unwired: 2 in, 2 out]
                }
                frame 81 {
                  n3193 = property on="Air Temperature  ( °C )" class="XYGraph (strict)"("Y Scale.Name Label.Text"=w4191) -> ()  [unwired: 2 in, 2 out]
                }
                frame 82 {
                  n3194 = local write "S 84"(w4192) -> ()
                }
                frame 83 {
                  n3195 = local write "S 85"(w4193) -> ()
                }
                frame 84 {
                  n3196 = local write "S 86"(w4194) -> ()
                }
                frame 85 {
                  n3197 = local write "S 87"(w4195) -> ()
                }
                frame 86 {
                  n3198 = local write "S 88"(w4196) -> ()
                }
                frame 87 {
                }
                frame 88 {
                  n3199 = local write "S 90"(w4198) -> ()
                }
                frame 89 {
                  n3200 = local write "S 91"(w4199) -> ()
                }
                frame 90 {
                  n3201 = local write "S 92"(w4200) -> ()
                }
                frame 91 {
                  n3202 = local write "S 93"(w4201) -> ()
                }
                frame 92 {
                  n3203 = local write "S 94"(w4202) -> ()
                }
                frame 93 {
                  n3204 = local write "S 95"(w4203) -> ()
                }
                frame 94 {
                  n3205 = local write "S 96"(w4204) -> ()
                }
                frame 95 {
                  n3206 = local write "S 97"(w4205) -> ()
                }
                frame 96 {
                  n3207 = local write "S 98"(w4206) -> ()
                }
                frame 97 {
                  n3208 = local write "S 99"(w4207) -> ()
                }
                frame 98 {
                  n3209 = local write "S 100"(w4208) -> ()
                }
                frame 99 {
                  n3210 = local write "S 101"(w4209) -> ()
                }
                frame 100 {
                  n3211 = local write "S 102"(w4210) -> ()
                }
                frame 101 {
                  n3212 = local write "S 103"(w4211) -> ()
                }
                frame 102 {
                  n3213 = local write "S 104"(w4212) -> ()
                }
                frame 103 {
                  n3214 = local write "S 105"(w4213) -> ()
                }
                frame 104 {
                  n3215 = local write "S 106"(w4214) -> ()
                }
                frame 105 {
                }
                frame 106 {
                  n3216 = property on="OK Button 17" class="Bool (strict)"("Boolean Text.Text"=w4215) -> ()  [unwired: 2 in, 2 out]
                }
                frame 107 {
                  n3217 = property on="OK Button 16" class="Bool (strict)"("Boolean Text.Text"=w4216) -> ()  [unwired: 2 in, 2 out]
                }
                frame 108 {
                  n3218 = property on="TITTLE" class="Str"("Caption.Text"=w4217) -> ()  [unwired: 2 in, 2 out]
                }
                frame 109 {
                  "String 30" <- w4218
                }
                frame 110 {
                  n3219 = property on="Test Date" class="Str"("Caption.Text"=w4219) -> ()  [unwired: 2 in, 2 out]
                  "String 31" <- w4219
                }
                frame 111 {
                  n3220 = property on="Sample ID" class="Str"("Caption.Text"=w4220) -> ()  [unwired: 2 in, 2 out]
                  "String 32" <- w4220
                }
                frame 112 {
                  n3221 = property on="Tested by" class="Str"("Caption.Text"=w4221) -> ()  [unwired: 2 in, 2 out]
                  "String 33" <- w4221
                }
                frame 113 {
                  n3222 = property on="System Configured Printers 2" class="Arr (strict)"("Caption.Text"=w4222) -> ()  [unwired: 2 in, 2 out]
                }
                frame 114 {
                  n3223 = property on="Selected Printer" class="Str"("Caption.Text"=w4223) -> ()  [unwired: 2 in, 2 out]
                }
                frame 115 {
                  n3224 = property on="Select Printer 3" class="DigNum (strict)"("Caption.Text"=w4224) -> ()  [unwired: 2 in, 2 out]
                }
                frame 116 {
                  n3225 = property on="Print" class="Bool (strict)"("Boolean Text.Text"=w4225) -> ()  [unwired: 2 in, 2 out]
                }
                frame 117 {
                  "String 41" <- w4226
                }
                frame 118 {
                  n3226 = property on="tested by" class="Str"("Caption.Text"=w4227) -> ()  [unwired: 2 in, 2 out]
                }
                frame 119 {
                }
                frame 120 {
                  n3227 = property on="Export" class="Bool (strict)"("Boolean Text.Text"=w4228) -> ()  [unwired: 2 in, 2 out]
                }
                frame 121 {
                }
                frame 122 {
                }
                frame 123 {
                  n3228 = property on="Select File Type" class="Enum (strict)"("Caption.Text"=w4231) -> ()  [unwired: 2 in, 2 out]
                }
                frame 124 {
                  n3229 = property on="s.NO" class="Str"("Caption.Text"=w4232) -> ()  [unwired: 2 in, 2 out]
                  "String 45" <- w4232
                }
                frame 125 {
                  n3230 = property on="trip1 8" class="Bool (strict)"("Boolean Text.Text"=w4233) -> ()  [unwired: 2 in, 2 out]
                }
                frame 126, Default {
                }
              }
            }
          }
          frame #1 {
            w4241 = TRUE ("Visible")
            n3231 = local read "S 91"() -> (w4258:string)
            n3232 = local read "S 90"() -> (w4257:string)
            n3233 = local read "S 88"() -> (w4256:string)
            n3234 = property on="File Path" class="Path"("Caption.Text"=w4257) -> ()  [unwired: 2 in, 2 out]
            n3235 = local read "S 71"() -> (w4251:string)
            n3236 = local read "S 86"() -> (w4253:string)
            n3237 = local read "S 85"() -> (w4254:string)
            n3238 = local read "S 87"() -> (w4252:string)
            n3239 = local read "S 84"() -> (w4255:string)
            n3240 = local read "S 103"() -> (w4240:string)
            n3241 = local read "S 104"() -> (w4239:string)
            n3242 = property on="Password" class="Str"("Caption.Text"=w4254) -> ()  [unwired: 2 in, 2 out]
            n3243 = property on="EDIT" class="Bool (strict)"("Boolean Text.Text"=w4251) -> ()  [unwired: 2 in, 2 out]
            n3244 = property on="SAVE" class="Bool (strict)"("Boolean Text.Text"=w4255) -> ()  [unwired: 2 in, 2 out]
            n3245 = Build Array(w4240, w4239) -> (w4238:string[])
            n3246 = property on="Heater Button" class="Bool (strict)"("Strings [4]"=w4238) -> ()  [unwired: 2 in, 2 out]
            n3247 = local read "S 92"() -> (w4250:string)
            n3248 = local read "S 93"() -> (w4249:string)
            n3249 = local read "S 105"() -> (w4236:string)
            n3250 = local read "S 106"() -> (w4235:string)
            n3251 = Build Array(w4250, w4249) -> ()  [unwired: 1 out]
            n3252 = Build Array(w4236, w4235) -> (w4237:string[])
            n3253 = local read "S 95"() -> (w4247:string)
            n3254 = local read "S 94"() -> (w4248:string)
            n3255 = local read "bs"() -> (w4263:string)
            n3256 = local read "as"() -> (w4264:string)
            n3257 = property on="Humidity" class="Bool (strict)"("Strings [4]"=w4237) -> ()  [unwired: 2 in, 2 out]
            n3258 = Concatenate Strings(w4263, "\r", w4264) -> ()  [unwired: 1 out]
            n3259 = property on="Rh After" class="DigNum (strict)"("Caption.Size to Text?"=TRUE ("Caption.Size to Text")) -> ()  [unwired: 2 in, 2 out]
            n3260 = local read "S 48"() -> (w4287:string)
            n3261 = local read "S 50"() -> (w4285:string)
            n3262 = local read "S 51"() -> (w4284:string)
            n3263 = local read "S 49"() -> (w4286:string)
            n3264 = local read "S 52"() -> (w4283:string)
            n3265 = local read "as"() -> (w4268:string)
            n3266 = local read "bs"() -> (w4269:string)
            n3267 = local read "S 56"() -> (w4282:string)
            n3268 = local read "S 57"() -> (w4281:string)
            n3269 = local read "S 58"() -> (w4280:string)
            n3270 = local read "S 59"() -> (w4279:string)
            n3271 = property on="OPEN" class="Bool (strict)"("Boolean Text.Text"=w4283) -> ()  [unwired: 2 in, 2 out]
            n3272 = property on="OPEN 1" class="Bool (strict)"("Boolean Text.Text"=w4287) -> ()  [unwired: 2 in, 2 out]
            n3273 = property on="OPEN 2" class="Bool (strict)"("Boolean Text.Text"=w4286) -> ()  [unwired: 2 in, 2 out]
            n3274 = property on="OPEN 3" class="Bool (strict)"("Boolean Text.Text"=w4285) -> ()  [unwired: 2 in, 2 out]
            n3275 = property on="OPEN 4" class="Bool (strict)"("Boolean Text.Text"=w4284) -> ()  [unwired: 2 in, 2 out]
            n3276 = Concatenate Strings(w4269, "\r", w4268) -> ()  [unwired: 1 out]
            n3277 = local read "S 102"() -> (w4242:string)
            n3278 = property on="КОФ1" class="DigNum (strict)"("Caption.Text"=w4282) -> ()  [unwired: 2 in, 2 out]
            n3279 = local read "S 98"() -> (w4246:string)
            n3280 = local read "S 99"() -> (w4245:string)
            n3281 = local read "S 100"() -> (w4244:string)
            n3282 = local read "S 101"() -> (w4243:string)
            n3283 = property on="КОФ2" class="DigNum (strict)"("Caption.Text"=w4281) -> ()  [unwired: 2 in, 2 out]
            n3284 = property on="КОФ3" class="DigNum (strict)"("Caption.Text"=w4280) -> ()  [unwired: 2 in, 2 out]
            n3285 = property on="КОФ4" class="DigNum (strict)"("Caption.Text"=w4279) -> ()  [unwired: 2 in, 2 out]
            n3286 = local read "bs"() -> (w4267:string)
            n3287 = local read "as"() -> (w4266:string)
            n3288 = local read "S 60"() -> (w4278:string)
            n3289 = local read "S 54"() -> (w4288:string)
            n3290 = Concatenate Strings(w4267, "\r", w4266) -> ()  [unwired: 1 out]
            n3291 = Concatenate Strings(w4288, w4278) -> ()  [unwired: 1 out]
            n3292 = local read "S 77"() -> (→"String 43":string)
            n3293 = local read "S 76"() -> (w4261:string)
            n3294 = local read "S 78"() -> (w4260:string)
            n3295 = local read "S 71"() -> (w4272:string)
            n3296 = local read "S 66"() -> (w4277:string)
            n3297 = local read "S 67"() -> (w4276:string)
            n3298 = local read "S 68"() -> (w4275:string)
            n3299 = local read "S 69"() -> (w4274:string)
            n3300 = local read "S 70"() -> (w4273:string)
            n3301 = property on="AIR TEMP" class="DigNum (strict)"("Caption.Text"=w4260) -> ()  [unwired: 2 in, 2 out]
            n3302 = property on="Set Strk" class="DigNum (strict)"("Caption.Text"=w4261) -> ()  [unwired: 2 in, 2 out]
            n3303 = property on="SPEED OUT:" class="DigNum (strict)"("Caption.Text"=w4275) -> ()  [unwired: 2 in, 2 out]
            n3304 = property on="EDIT" class="Bool (strict)"("Boolean Text.Text"=w4272) -> ()  [unwired: 2 in, 2 out]
            n3305 = local read "S 79"() -> (w4259:string)
          }
          frame #2 {
          }
        }
        n3306 = local write "Lan flag"(10.0 ("Lan flag")) -> ()
      }
      frame Enabled {
      }
    }
    n3307 = Wait (ms)(milliseconds to wait=u32 2000) -> ()  [unwired: 1 out]
    n3308 = local read "Quit"() -> (w4062:bool)
  }
  n3309 = while {
    shift-right: [w4294] -> _
    shift-left: _ -> [w4295]
    shift-right: [w4292] -> _
    shift-left: T18 {"Read Heave and Surge"="", "Bytes at Heave Port"=0.0, "Heave and Surge COM Port:"="COM9", "Com Port 2"="COM7", "Residual Due"="", "Heave COM Status 2"=TRUE, "Heave COM Status"=TRUE, "Port 2"=TRUE, "Sway PPR"=6400.0, "Surge PPR"=6400.0, "Heave PPR"=6400.0, "Sway Pitch"=2.0, "Surge Pitch"=3.0, "Heave Pitch"=4.0, "Sway Pulses/mm"=320.0, "Surge Pulses/mm"=1600.0, "Heave Pulses/mm"=1600.0, "inner loop"=0.0, "Read Heave and Surge 2"="", "String 36"="", "Write S"=FALSE, "WriteCC1"=[""], "Heave COM Loop"=0, "LastCom"="", "EXIT"=FALSE, "Error Heave"={"status"=TRUE, "code"=-1073807343, "source"=""}} -> [w4291]
    shift-right: [w4289] -> _
    shift-left: enum16{"init", "MAIN", "Panel Close"}."init" -> [w4290]
    stop <- w4293 stop-if-true
    # "HUMIDITY LOOP LOGIC"
    n3310 = case shown="\"MAIN\"" w4290 {
      tunnel: w4295 -> [w4309 w4328 w4383 w4385]
      tunnel: [w4304 w4332 w4383 w4385] -> w4294
      tunnel: [_ _ TRUE _] -> w4293
      tunnel: [w4301 w4330 w4381 w4384] -> w4292
      tunnel: w4291 -> [w4306 w4327 w4381 w4384]
      tunnel: [enum16{"init", "MAIN", "Panel Close"}."MAIN" w4322 _ _] -> w4289
      frame "init" {
        n3311 = local read "C3 :"() -> (w4296:refnum<visa-resource-name>)
        n3312 = Bundle By Name(cluster=w4306, "Heave and Surge COM Port:"=w4296) -> (w4305:T18)
        n3313 = call "Instrument fgv uno.vi"("Enum"=T31."INIT", "error in (no error) 2"=w4309, "INPUT"=w4305) -> ("error"=w4307:errorcluster, "output"=w4303:T18)  [unwired: 6 in, 1 out]
        n3314 = case shown="Error" w4307 {
          selector: w4307 -> [w4311 _]
          tunnel: [w4311 w4315] -> w4304
          tunnel: w4303 -> [w4310 w4313]
          tunnel: [w4310 w4312] -> w4302
          frame No Error {
          }
          frame Error {
            n3315 = call "Instrument fgv uno.vi"("Enum"=T31."ERROR INIT", "INPUT"=w4313) -> ("error"=w4316:errorcluster, "output"=w4312:T18)  [unwired: 7 in, 1 out]
            n3316 = call <vilib>:"Clear Errors.vi"("error in (no error)"=w4316) -> ("error out"=w4315:errorcluster)  [unwired: 5 in, 1 out]
          }
        }
        n3317 = local read "LastCom Humidity"() -> (w4299:string)
        n3318 = Unbundle By Name(w4302) -> ("Heave COM Status 2"=→"COM Status":bool, "Error Heave"=→"Error":errorcluster)  [unwired: 1 out]
        n3319 = Bundle By Name(cluster=w4302, "LastCom"=w4299) -> (w4301:T18)
      }
      frame "MAIN" {
        n3320 = Unbundle By Name(w4327) -> ("Com Port 2"=w4317:refnum<visa-resource-name>)
        n3321 = local read "C3 :"() -> (w4318:refnum<visa-resource-name>)
        n3322 = local write "COM Port Humidity :"(w4317) -> ()
        n3323 = Bundle By Name(cluster=w4327, "Heave and Surge COM Port:"=w4318) -> (w4326:T18)
        n3324 = Equal?(x=w4317, y=w4318) -> (x = y?=w4333:bool)
        n3325 = case shown="True" w4333 {
          tunnel: [w4337 w4354] -> w4332
          tunnel: w4328 -> [w4338 w4360]
          tunnel: w4326 -> [w4336 w4358]
          tunnel: [w4335 w4353] -> w4330
          frame False {
            n3326 = call <vilib>:"Clear Errors.vi"("error in (no error)"=w4338) -> ("error out"=w4334:errorcluster)  [unwired: 5 in, 1 out]
            n3327 = call "Instrument fgv uno.vi"("Enum"=T31."ERROR INIT", "error in (no error) 2"=w4334, "INPUT"=w4336) -> ("error"=w4340:errorcluster, "output"=w4335:T18)  [unwired: 6 in, 1 out]
            n3328 = call <vilib>:"Clear Errors.vi"("error in (no error)"=w4340) -> ("error out"=w4337:errorcluster)  [unwired: 5 in, 1 out]
          }
          frame True {
            n3329 = call "Instrument fgv uno.vi"("Enum"=T31."READ", "error in (no error) 2"=w4360, "INPUT"=w4358) -> ("error"=w4359:errorcluster, "output"=w4352:T18)  [unwired: 6 in, 1 out]
            n3330 = Bundle By Name(cluster=w4352, "String 36"="WRITE HUMIDITY") -> (w4351:T18)
            n3331 = case shown="True" "Write Humidity" {
              selector: "Write Humidity" -> [_ w4380]
              tunnel: w4359 -> [w4373 w4379]
              tunnel: [w4373 w4378] -> w4349
              tunnel: w4351 -> [w4372 w4376]
              tunnel: [w4372 w4375] -> w4348
              frame False {
              }
              frame True {
                n3332 = Not(x=w4380) -> (.not. x?=w4374:bool)
                n3333 = local write "Write Humidity"(w4374) -> ()
                n3334 = call "Instrument fgv uno.vi"("Enum"=T31."MANUAL WRITE", "error in (no error) 2"=w4379, "INPUT"=w4376) -> ("error"=w4378:errorcluster, "output"=w4375:T18)  [unwired: 6 in, 1 out]
              }
            }
            n3335 = Array Size(array="WriteHumidity") -> (size(s)=w4346:i32)
            n3336 = Greater Than 0?(x=w4346) -> (x > 0?=w4345:bool)
            n3337 = call "Instrument fgv uno.vi"("Enum"=T31."WRITE", "error in (no error) 2"=w4349, "WriteCC1"="WriteHumidity", "INPUT"=w4348) -> ("error"=w4356:errorcluster, "WriteCC1 2"=w4347:string[], "output"=w4355:T18)  [unwired: 5 in]
            n3338 = case shown="True" w4345 {
              tunnel: w4347 -> [_ w4362]
              frame False {
              }
              frame True {
                n3339 = local write "WriteHumidity"(w4362) -> ()
              }
            }
            n3340 = case shown="No Error" w4356 {
              selector: w4356 -> [w4363 w4366]
              tunnel: w4355 -> [w4364 w4371]
              tunnel: [w4364 w4370] -> w4353
              tunnel: [w4363 w4368] -> w4354
              frame No Error {
              }
              frame Error {
                n3341 = call <vilib>:"Clear Errors.vi"("error in (no error)"=w4366) -> ("error out"=w4365:errorcluster)  [unwired: 5 in, 1 out]
                n3342 = call "Instrument fgv uno.vi"("Enum"=T31."ERROR INIT", "error in (no error) 2"=w4365, "INPUT"=w4371) -> ("error"=w4369:errorcluster, "output"=w4370:T18)  [unwired: 6 in, 1 out]
                n3343 = call <vilib>:"Clear Errors.vi"("error in (no error)"=w4369) -> ("error out"=w4368:errorcluster)  [unwired: 5 in, 1 out]
              }
            }
            n3344 = Unbundle By Name(w4353) -> ("LastCom"=→"LastCom Humidity":string, "Read Heave and Surge"=→"Read HUMIDITY":string)
          }
        }
        n3345 = Unbundle By Name(w4330) -> ("Heave COM Status 2"=w4331:bool, "Error Heave"=w4319:errorcluster, "Bytes at Heave Port"=→"Bytes at Humidity Port  2":dbl)  [unwired: 1 out]
        n3346 = Unbundle By Name(w4319) -> ("status"=→"Humidity Port":bool)
        n3347 = Not(x=w4331) -> (.not. x?=w4320:bool)
        n3348 = local write "Error"(w4319) -> ()
        n3349 = local read "Quit"() -> (w4323:bool)
        n3350 = local write "COM Status"(w4320) -> ()
        n3351 = Select(t=enum16{"init", "MAIN", "Panel Close"}."Panel Close", s=w4323, f=enum16{"init", "MAIN", "Panel Close"}."MAIN") -> (s? t:f=w4322:enum16{"init", "MAIN", "Panel Close"})
      }
      frame "Panel Close" {
      }
      frame Default {
      }
    }
  }
  n3352 = while {
    shift-right: [w4391] -> _
    shift-left: _ -> [w4392]
    shift-right: [w4389] -> _
    shift-left: T20 {"Read Uno"="", "Bytes at Heave Port"=0.0, "UNO COM Port:"="COM9", "UNO COM Port: 2"="COM7", "Residual Due"="", "UNO COM Status 2"=TRUE, "UNO COM Status"=TRUE, "Port 2"=TRUE, "Sway PPR"=6400.0, "Surge PPR"=6400.0, "Heave PPR"=6400.0, "Sway Pitch"=2.0, "Surge Pitch"=3.0, "Heave Pitch"=4.0, "Sway Pulses/mm"=320.0, "Surge Pulses/mm"=1600.0, "Heave Pulses/mm"=1600.0, "inner loop"=0.0, "Read Heave and Surge 2"="", "String 36"="", "Write S"=FALSE, "WriteCC1"=[""], "Heave COM Loop"=0, "LastCom"="", "EXIT"=FALSE, "Error Heave"={"status"=TRUE, "code"=-1073807343, "source"=""}} -> [w4388]
    shift-right: [w4386] -> _
    shift-left: enum16{"init", "MAIN", "Panel Close"}."init" -> [w4387]
    stop <- w4390 stop-if-true
    # "UNO CODE LOGIC"
    n3353 = case shown="\"MAIN\"" w4387 {
      tunnel: w4392 -> [w4406 w4425 w4481 w4483]
      tunnel: [w4401 w4430 w4481 w4483] -> w4391
      tunnel: [_ _ TRUE _] -> w4390
      tunnel: [w4397 w4428 w4479 w4482] -> w4389
      tunnel: w4388 -> [w4403 w4424 w4479 w4482]
      tunnel: [enum16{"init", "MAIN", "Panel Close"}."MAIN" w4419 _ _] -> w4386
      frame "init" {
        n3354 = local read "Com Port 1"() -> (w4393:refnum<visa-resource-name>)
        n3355 = Bundle By Name(cluster=w4403, "UNO COM Port:"=w4393) -> (w4402:T20)
